vi "一体站流程质控自动启动.vi"(6 "CODMn量程切换":enum32{"H", "L", "AUTO"}(ring)=enum."AUTO", 8 "总磷量程切换":enum32{"H", "L", "AUTO"}(ring)=enum."AUTO", 9 "总氮量程切换":enum32{"H", "L", "AUTO"}(ring)=enum."AUTO", 10 "氨氮量程切换":enum32{"H", "L", "AUTO"}(ring)=enum."AUTO", 11 "参数":T1={"是否启用仪器"=FALSE, "CODMn"={"启动测量模式"={"测量模式"=enum."水样测量"}, "确定按钮"=TRUE}, "启动模块"={"氨氮"=FALSE, "总磷"=FALSE, "总氮"=FALSE, "COD"=FALSE}, "常规启动"=FALSE, "直接启动"=FALSE}) -> ()   [LabVIEW 2016, in "质控单元.lvlib"]
uses:
  PLC/PLC.lvlib
panel:
  out "枚举 2":enum16{"初始化", "采配水启动", "等待", "配水", "排水", "结束"}(ring)
  out "枚举":enum16{"初始化", "采配水启动", "等待", "配水", "排水", "结束"}(ring)
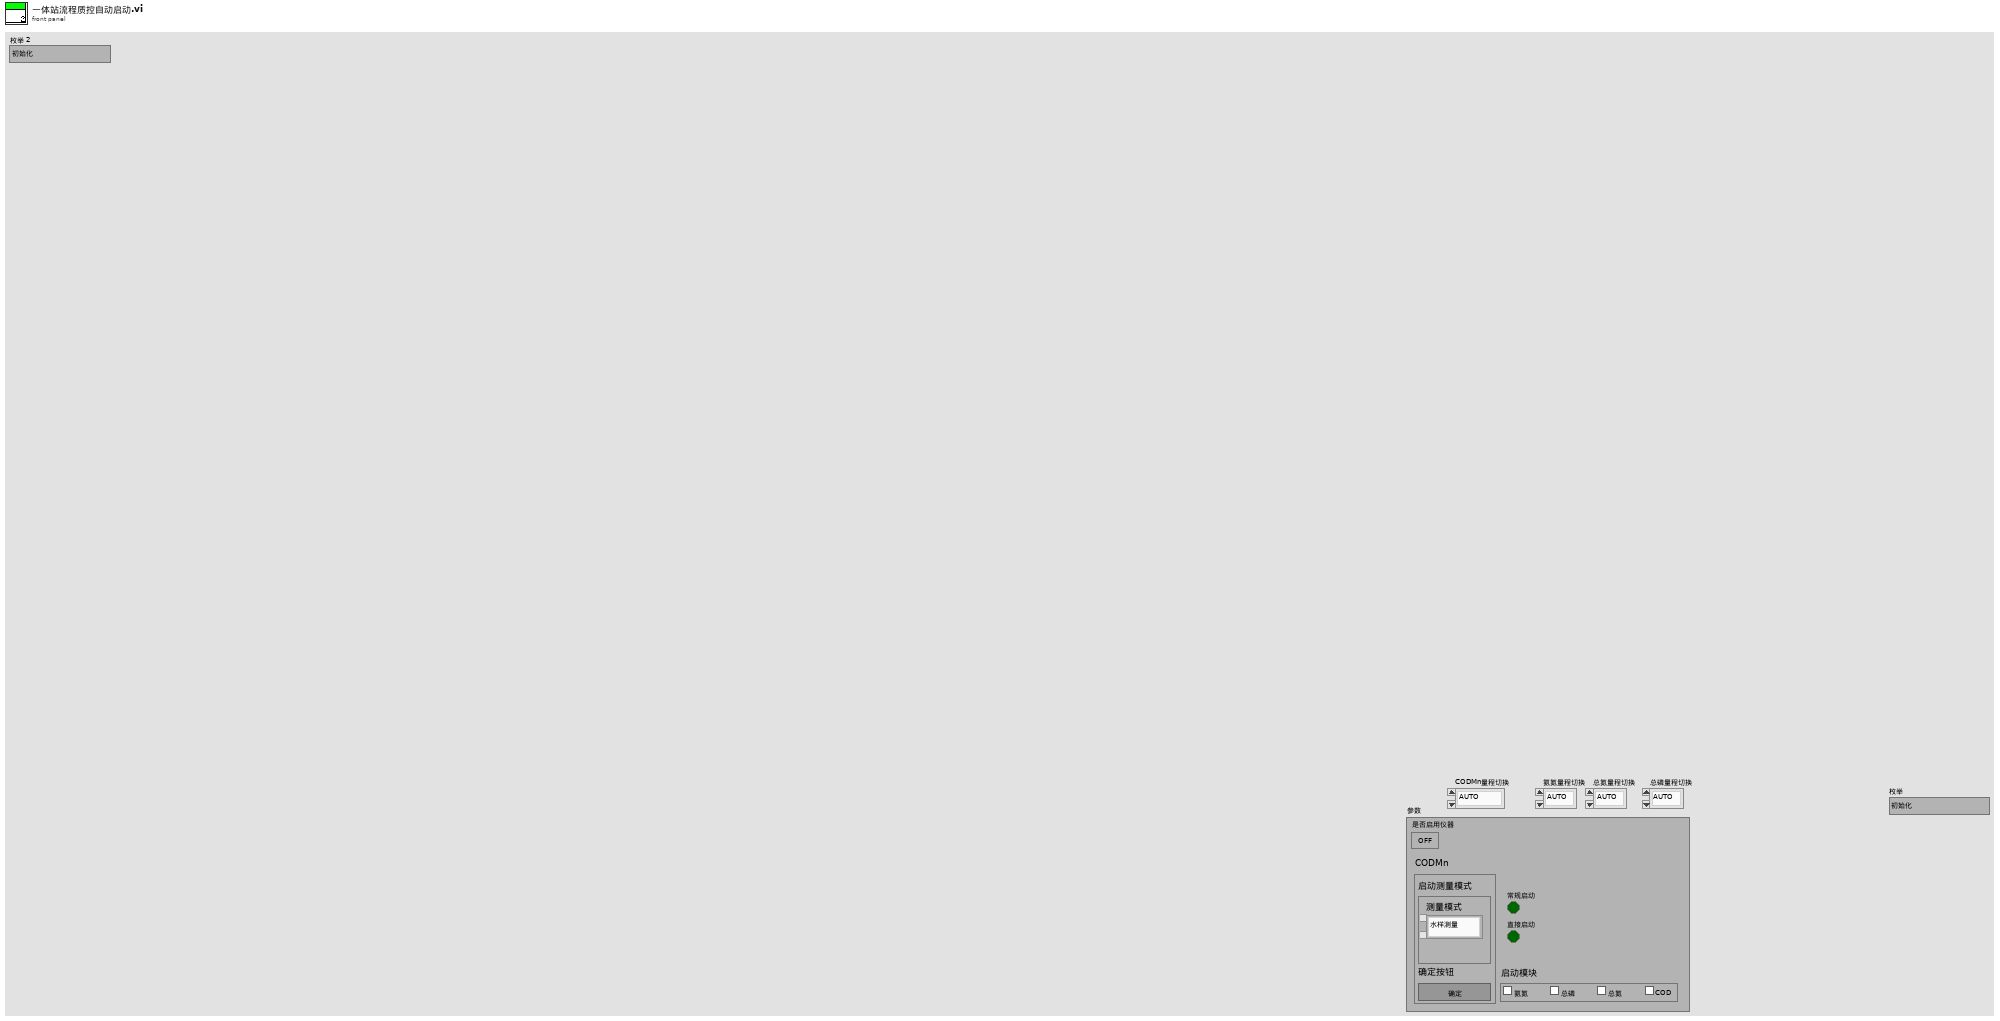
[diagram p1: front panel]
types:
  T1 = cluster{"是否启用仪器":bool, "CODMn":cluster{"启动测量模式":cluster{"测量模式":enum16{"水样测量", "标样核查", "加标回收", "平行样", "校零", "校标"}}, "确定按钮":bool}, "启动模块":cluster{"氨氮":bool, "总磷":bool, "总氮":bool, "COD":bool}, "常规启动":bool, "直接启动":bool}
  T2 = cluster{"命令":string, cluster{"starting address":u16, "holding register value":u16}}
  T3 = cluster{"R0":i16, "R1":i16, "R2":i16, "R3":i16, "R4":i16, "R5":i16, "R6":i16, "R7":i16, "R8":i16, "R9":i16, "R10":i16, "R11":i16, "R12":i16, "R13":i16, "R14":i16, "R15":i16, "R16":i16, "R17":i16, "R18":i16, "R19":i16, "R20":i16, "R21":i16, "R22":i16, "R23":i16, "R24":i16, "R25":i16, "R26":i16, "R27":i16, "R28":i16, "R29":i16, "R30":i16, "R31":i16, "R32":i16, "R33":i16, "R34":i16, "R35":i16, "R36":i16, "R37":i16, "R38":i16, "R39":i16, "R40":i16, "R41":i16, "R42":i16, "R43":i16, "R44":i16, "R45":i16, "R46":i16, "R47":i16, "R48":i16, "R49":i16, "R50":i16, "R51":i16, "R52":i16, "R53":i16, "R54":i16, "R55":i16, "R56":i16}
  T4 = enum32{"Bad", "Idle", "Run top level", "Running"}
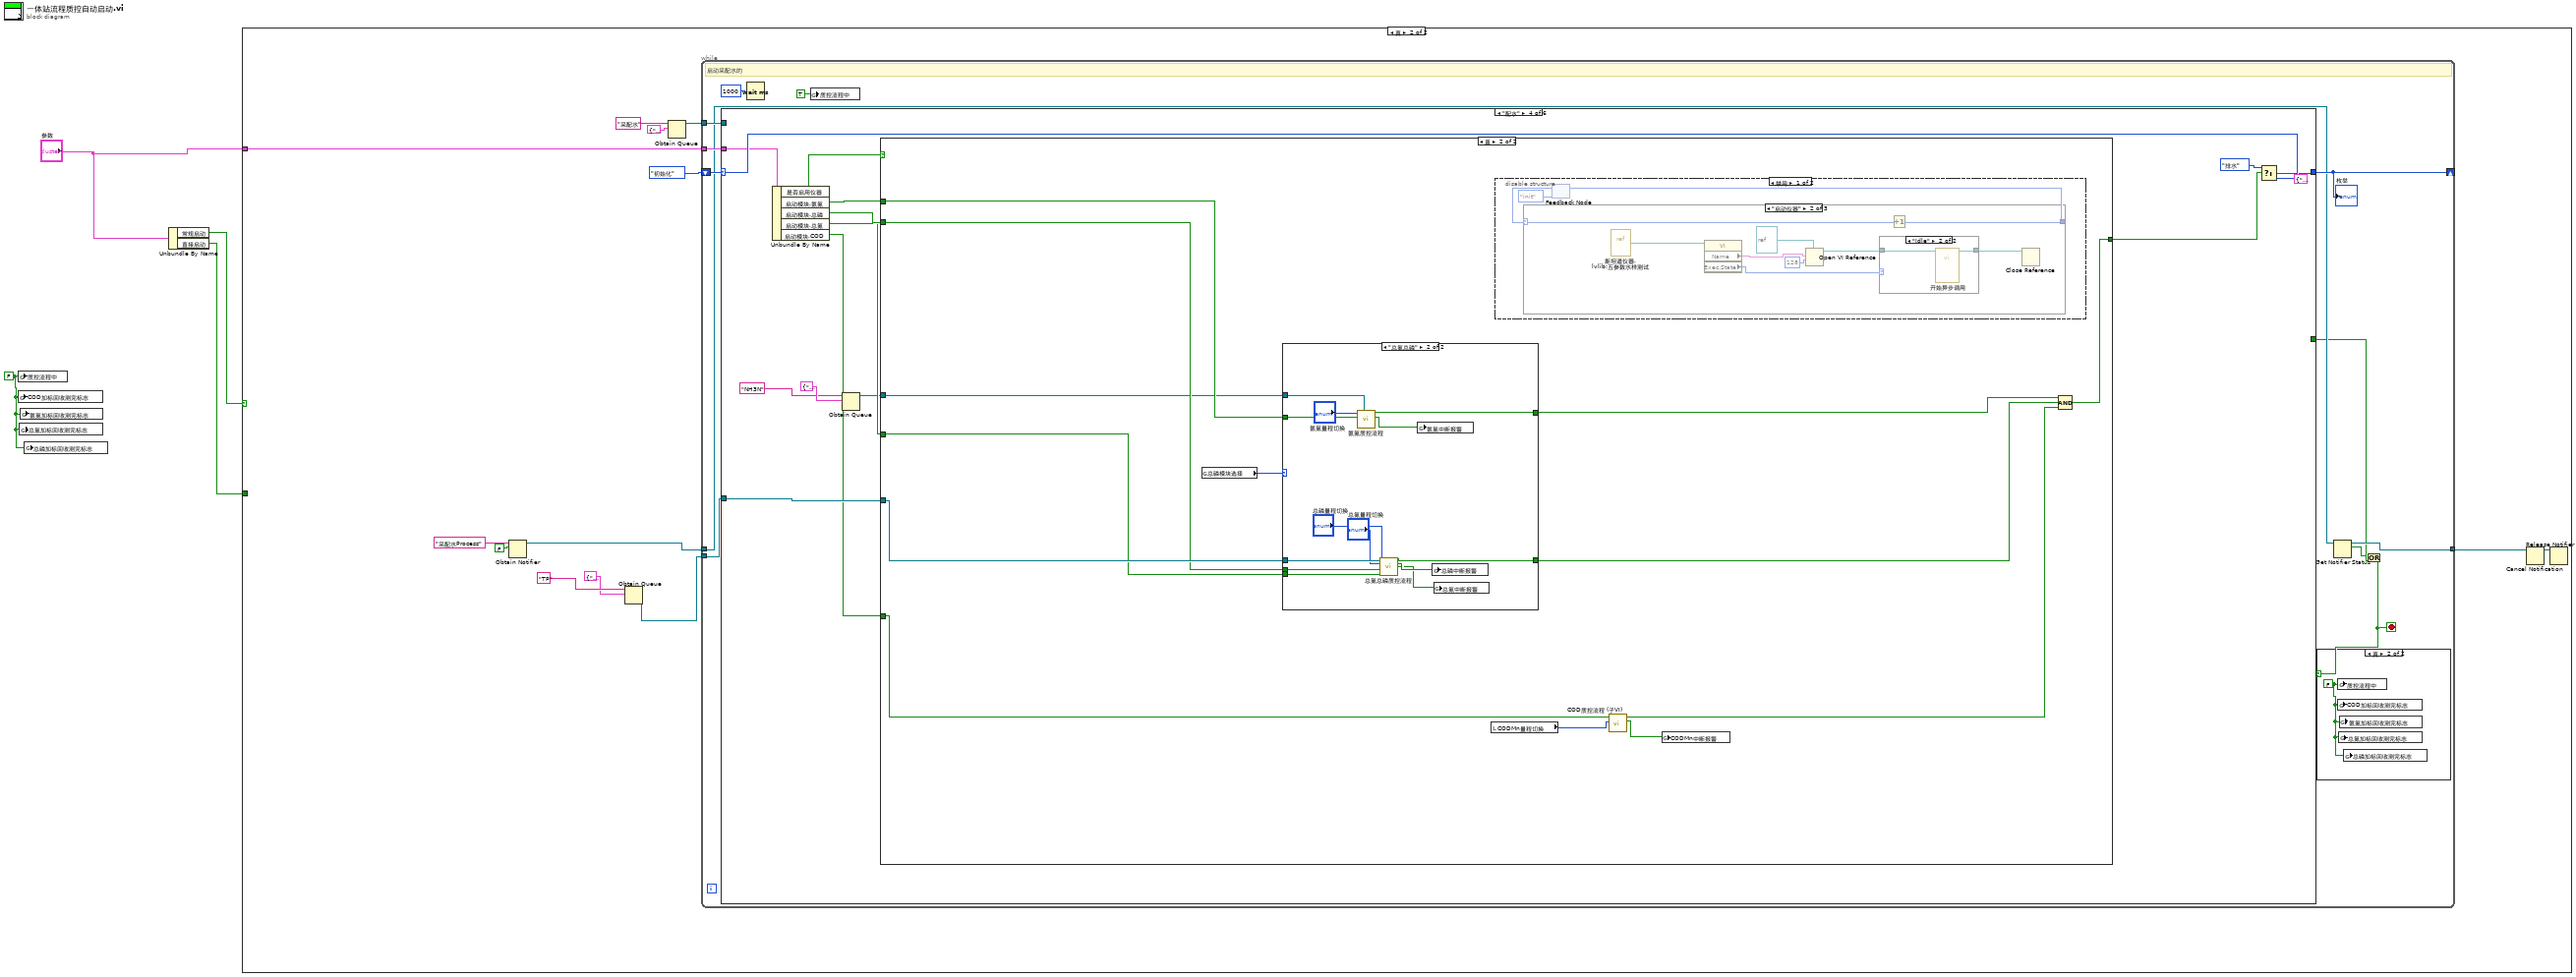
[diagram p0: block diagram]
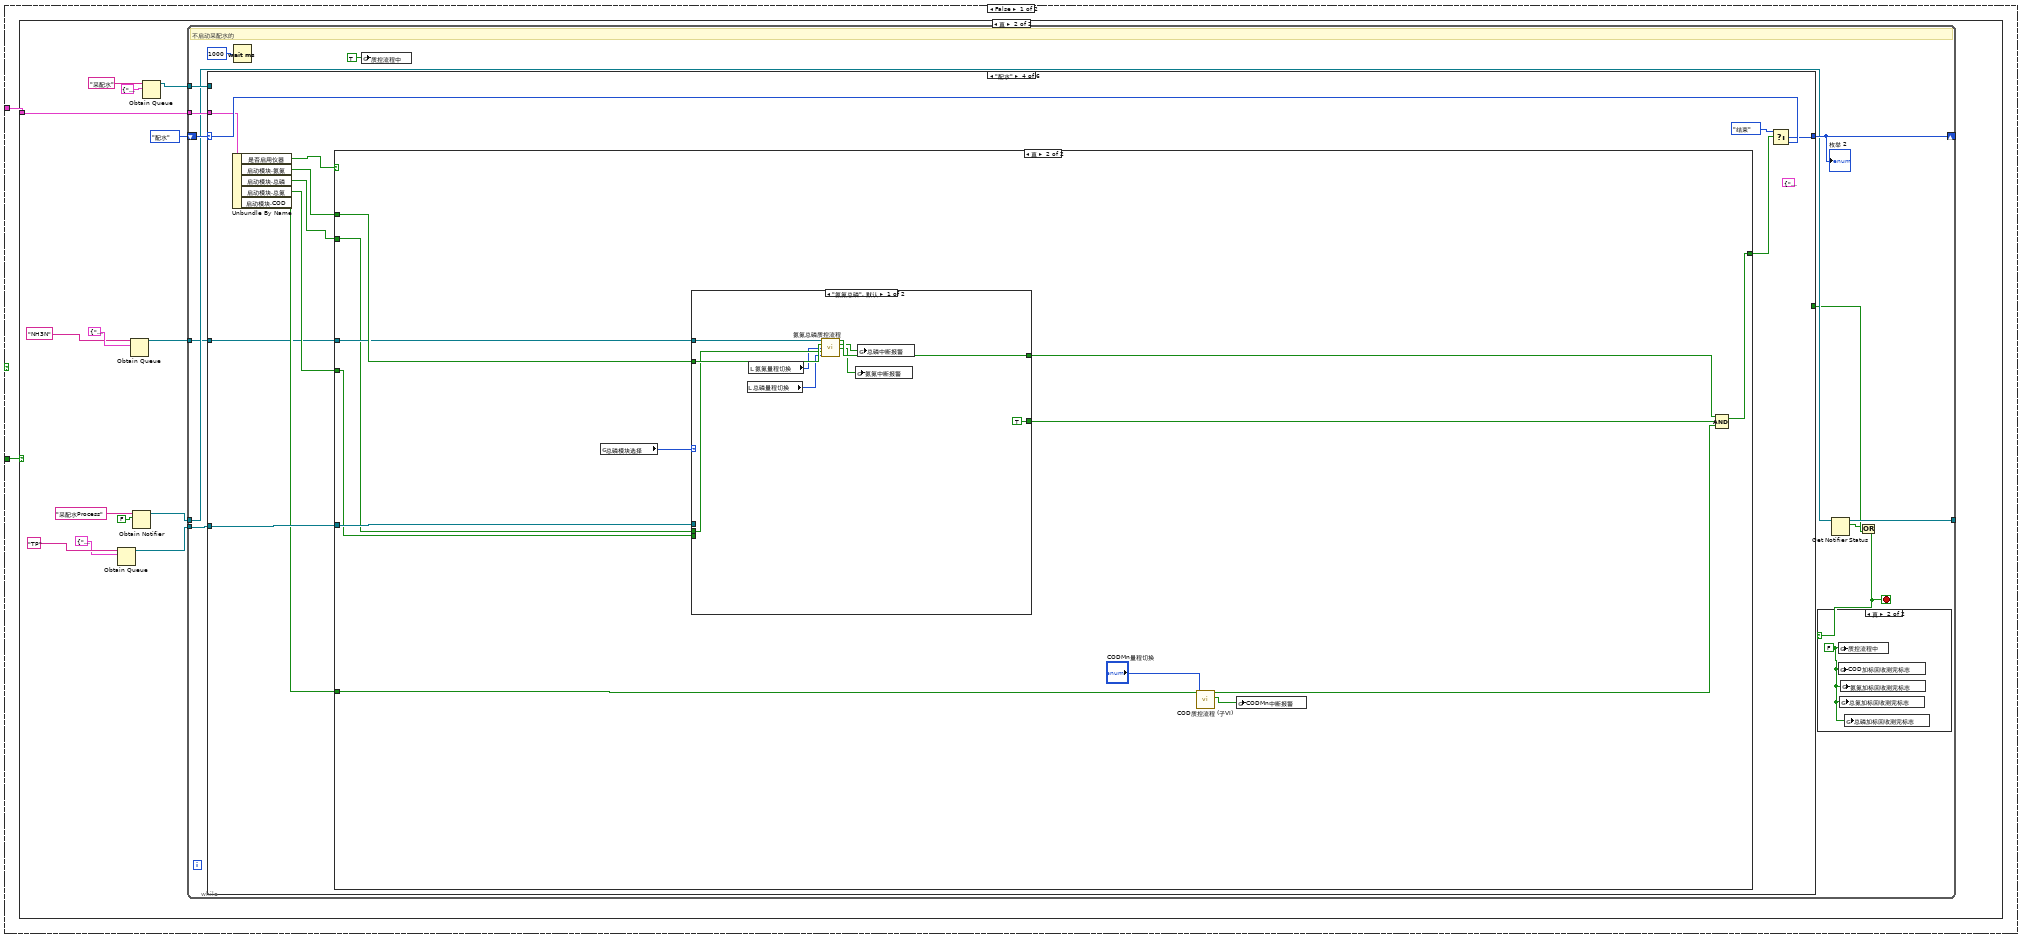
[diagram p2: hidden frame]
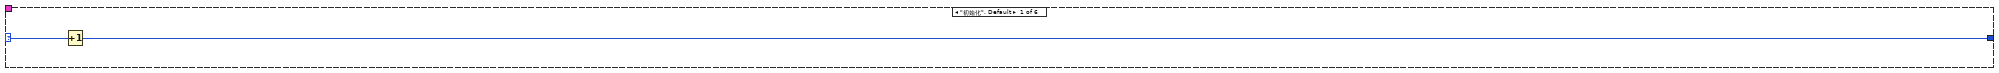
[diagram p5: hidden frame]
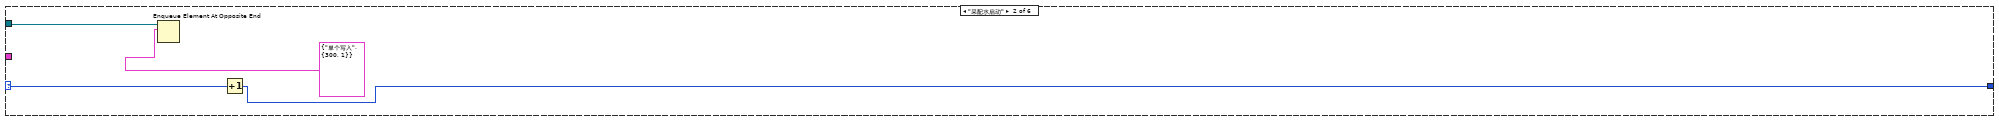
[diagram p6: hidden frame]
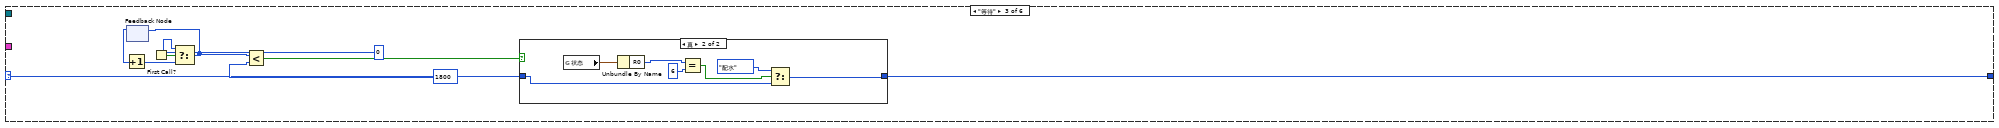
[diagram p7: hidden frame]
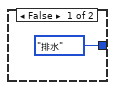
[diagram p8: hidden frame]
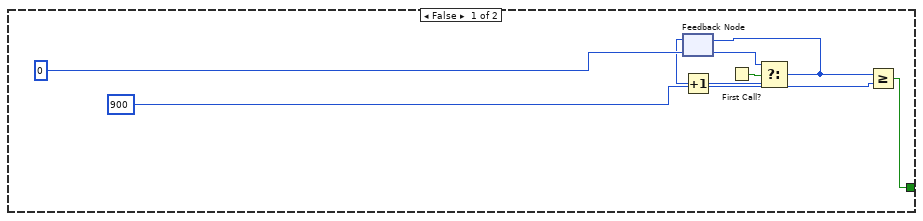
[diagram p9: hidden frame]
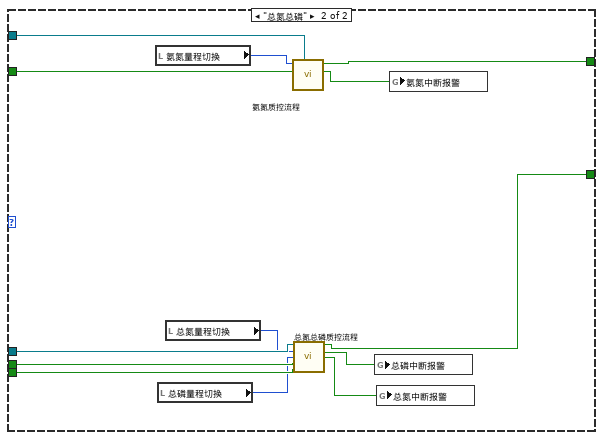
[diagram p10: hidden frame]
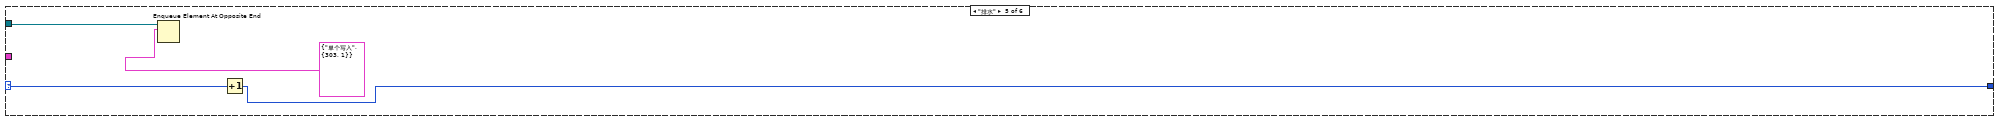
[diagram p11: hidden frame]
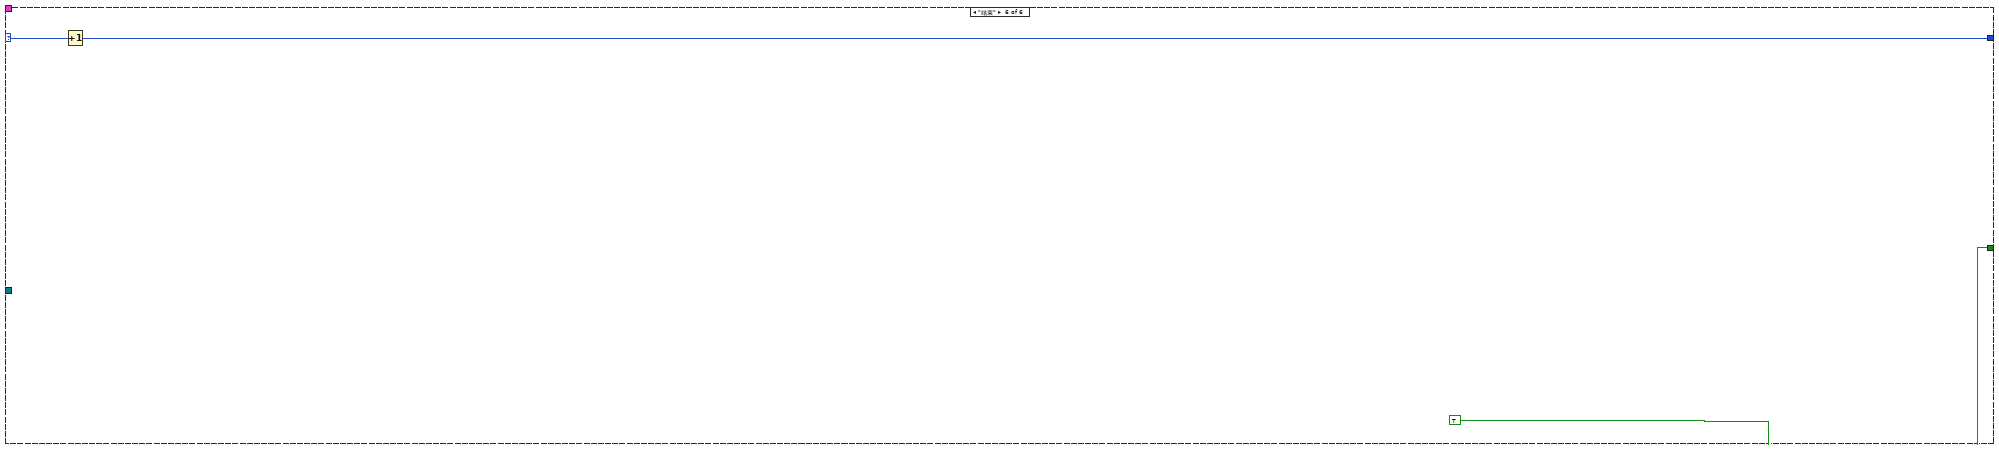
[diagram p12: hidden frame]
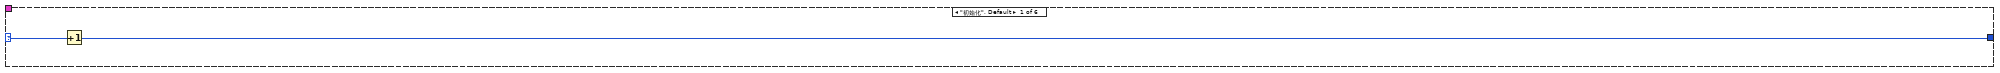
[diagram p14: hidden frame]
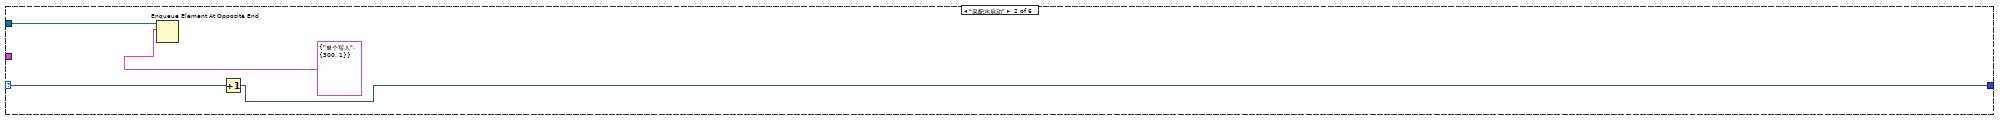
[diagram p15: hidden frame]
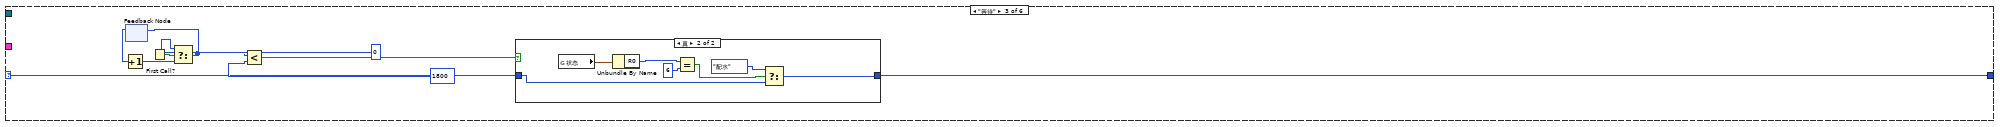
[diagram p16: hidden frame]
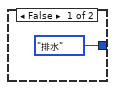
[diagram p17: hidden frame]
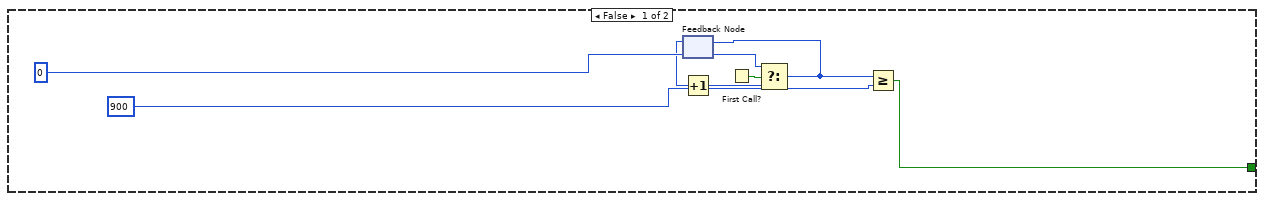
[diagram p18: hidden frame]
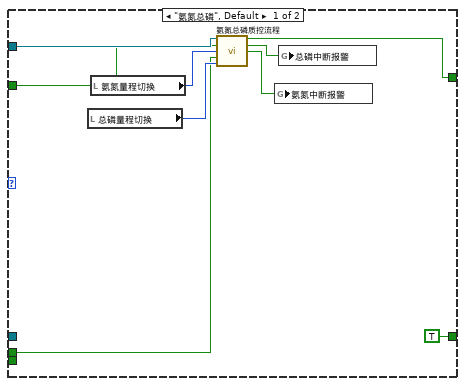
[diagram p19: hidden frame]
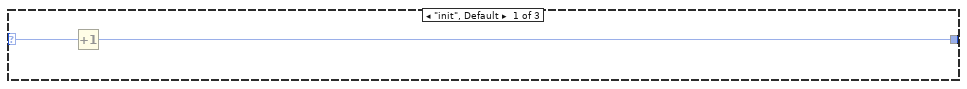
[diagram p20: hidden frame]
diagram:
  w1 = FALSE ("质控流程中")
  n1 = global write "质控测完标志全局 1.vi" "质控流程中"(w1) -> ()
  n2 = global write "质控测完标志全局 1.vi" "COD加标回收测完标志"(w1) -> ()
  n3 = global write "质控测完标志全局 1.vi" "总氮加标回收测完标志"(w1) -> ()
  n4 = global write "质控测完标志全局 1.vi" "氨氮加标回收测完标志"(w1) -> ()
  n5 = global write "质控测完标志全局 1.vi" "总磷加标回收测完标志"(w1) -> ()
  n6 = Unbundle By Name("参数") -> ("常规启动"=w3:bool, "直接启动"=w2:bool)
  n7 = case shown="真" w3 {
    tunnel: "参数" -> [w5 w119]
    tunnel: w2 -> [w6 _]
    frame False {
      n8 = case shown="真" w6 {
        tunnel: w5 -> [_ w19]
        frame False {
        }
        frame True {
          n9 = Obtain Queue(name (unnamed)="TP" ("名称（未命名）"), element data type=cluster{"命令":string, "data":variant} {"命令"="", "data"=variant}) -> (queue out=w10:refnum<queue>)  [unwired: 3 in, 2 out]
          n10 = Obtain Queue(name (unnamed)="NH3N" ("名称（未命名）"), element data type=cluster{"命令":string, "data":variant} {"命令"="", "data"=variant}) -> (queue out=w7:refnum<queue>)  [unwired: 3 in, 2 out]
          n11 = Obtain Notifier(name (unnamed)="采配水Process" ("名称（未命名）"), notification data type=FALSE) -> (notifier out=w13:refnum<notifier>)  [unwired: 2 in, 2 out]
          n12 = Obtain Queue(name (unnamed)="采配水" ("名称（未命名）"), element data type=cluster{"命令":string, "数据":variant} {"命令"="", "数据"=variant}) -> (queue out=w16:refnum<queue>)  [unwired: 3 in, 2 out]
          n13 = while {
            tunnel: w16 -> [w33]
            shift-right: [w31] -> _
            shift-left: enum16{"初始化", "采配水启动", "等待", "配水", "排水", "结束"}."配水" ("枚举") -> [w32]
            tunnel: w10 -> [w29]
            tunnel: w19 -> [w28]
            tunnel: w13 -> [w27]
            tunnel: [w26] -> _
            tunnel: w7 -> [w23]
            stop <- w22 stop-if-true
            # "不启动采配水的"
            n14 = case shown="\"配水\"" w32 {
              selector: w32 -> [w36 w38 w47 w68 w113 w118]
              tunnel: w33 -> [_ w39 _ _ w114 _]
              tunnel: [w35 w37 w46 w67 w112 w117] -> w31
              tunnel: [_ _ _ _ _ TRUE] -> w25
              tunnel: w29 -> [_ _ _ w66 _ _]
              tunnel: w28 -> [_ _ _ w63 _ _]
              tunnel: w23 -> [_ _ _ w58 _ _]
              frame "初始化", Default {
                n15 = Increment(x=w36) -> (x+1=w35:enum16{"初始化", "采配水启动", "等待", "配水", "排水", "结束"})
              }
              frame "采配水启动" {
                n16 = Enqueue Element At Opposite End(queue=w39, element=T2 {"命令"="单个写入", {"starting address"=300, "holding register value"=1}} ("元素")) -> ()  [unwired: 2 in, 3 out]
                n17 = Increment(x=w38) -> (x+1=w37:enum16{"初始化", "采配水启动", "等待", "配水", "排水", "结束"})
              }
              frame "等待" {
                n18 = feedback #1() -> (w43:i32)  [unwired: 1 in]
                n19 = Increment(x=w43) -> (x+1=w42:i32)
                n20 = First Call?() -> (First Call?: T/F=w44:bool)
                n21 = Select(t=0, s=w44, f=w42) -> (s? t:f=w41:i32)
                n22 = feedback-in #1(w41) -> ()
                n23 = Less?(x=w41, y=1800) -> (x < y?=w48:bool)
                n24 = case shown="真" w48 {
                  tunnel: w47 -> [_ w52]
                  tunnel: [enum16{"初始化", "采配水启动", "等待", "配水", "排水", "结束"}."排水" ("枚举") w51] -> w46
                  frame False {
                  }
                  frame True {
                    n25 = global read "采配水全局变量.vi" "状态"() -> (w57:T3)
                    n26 = Unbundle By Name(w57) -> ("R0"=w56:i16)
                    n27 = Equal?(x=w56, y=i16 6) -> (x = y?=w54:bool)
                    n28 = Select(t=enum16{"初始化", "采配水启动", "等待", "配水", "排水", "结束"}."配水" ("枚举"), s=w54, f=w52) -> (s? t:f=w51:enum16{"初始化", "采配水启动", "等待", "配水", "排水", "结束"})
                  }
                }
              }
              frame "配水" {
                (unwired) cluster{"命令":string, "data":variant} {"命令"="启动", "data"=variant(cluster{"站号":u16, "控制命令输出":u16[]} {"站号"=1, "控制命令输出"=[256, 0]})} ("元素")
                n29 = Unbundle By Name(w63) -> ("是否启用仪器"=w65:bool, "启动模块.氨氮"=w61:bool, "启动模块.总磷"=w62:bool, "启动模块.总氮"=w59:bool, "启动模块.COD"=w60:bool)
                n30 = case shown="真" w65 {
                  tunnel: w66 -> [_ w83]
                  tunnel: [w70 w89] -> w64
                  tunnel: w62 -> [_ w82]
                  tunnel: w61 -> [_ w88]
                  tunnel: w60 -> [_ w87]
                  tunnel: w59 -> [_ w81]
                  tunnel: w58 -> [_ w85]
                  frame False {
                    n31 = feedback #2() -> (w74:i32)  [unwired: 1 in]
                    n32 = Increment(x=w74) -> (x+1=w73:i32)
                    n33 = First Call?() -> (First Call?: T/F=w75:bool)
                    n34 = Select(t=0, s=w75, f=w73) -> (s? t:f=w71:i32)
                    n35 = feedback-in #2(w71) -> ()
                    n36 = Greater Or Equal?(x=w71, y=900) -> (x >= y?=w70:bool)
                  }
                  frame True {
                    n37 = global read "质控测完标志全局 1.vi" "总磷模块选择"() -> (w77:enum32{"氨氮总磷", "总氮总磷"})
                    n38 = case shown="\"氨氮总磷\", 默认" w77 {
                      tunnel: w88 -> [w96 w111]
                      tunnel: [w92 w110] -> w86
                      tunnel: w85 -> [w97 w109]
                      tunnel: w83 -> [_ w108]
                      tunnel: w82 -> [w95 w107]
                      tunnel: w81 -> [_ w106]
                      tunnel: [TRUE ("布尔") w105] -> w80
                      frame "氨氮总磷", Default {
                        n39 = local read "总磷量程切换"() -> (w93:enum32{"H", "L", "AUTO"})
                        n40 = local read "氨氮量程切换"() -> (w94:enum32{"H", "L", "AUTO"})
                        n41 = call "氨氮总磷质控流程.vi"("队列输入"=w97, "氨氮"=w96, "氨氮量程切换"=w94, "总磷"=w95, "总磷量程切换"=w93) -> ("布尔"=w92:bool, "总磷中断报警"=w91:bool, "氨氮中断报警"=w90:bool)  [unwired: 8 in]
                        n42 = global write "质控中断报警全局.vi" "氨氮中断报警"(w90) -> ()
                        n43 = global write "质控中断报警全局.vi" "总磷中断报警"(w91) -> ()
                      }
                      frame "总氮总磷" {
                        n44 = local read "氨氮量程切换"() -> (w102:enum32{"H", "L", "AUTO"})
                        n45 = local read "总磷量程切换"() -> (w104:enum32{"H", "L", "AUTO"})
                        n46 = local read "总氮量程切换"() -> (w103:enum32{"H", "L", "AUTO"})
                        n47 = call "氨氮质控流程.vi"("队列输入NH3"=w109, "氨氮"=w111, "氨氮量程切换"=w102) -> ("氨氮中断报警"=w101:bool, "布尔"=w110:bool)  [unwired: 7 in]
                        n48 = call "总氮总磷质控流程.vi"("队列输入TP"=w108, "总氮量程切换"=w103, "总磷量程切换"=w104, "总磷"=w107, "总氮"=w106) -> ("布尔"=w105:bool, "总磷中断报警"=w100:bool, "总氮中断报警"=w99:bool)  [unwired: 8 in]
                        n49 = global write "质控中断报警全局.vi" "总磷中断报警"(w100) -> ()
                        n50 = global write "质控中断报警全局.vi" "总氮中断报警"(w99) -> ()
                        n51 = global write "质控中断报警全局.vi" "氨氮中断报警"(w101) -> ()
                      }
                    }
                    n52 = call "COD质控流程 (子VI).vi"("CODMn量程切换"="CODMn量程切换", "COD"=w87) -> ("CODMn中断报警"=w78:bool, "布尔"=w84:bool)  [unwired: 8 in]
                    n53 = global write "质控中断报警全局.vi" "CODMn中断报警"(w78) -> ()
                    n54 = Compound Arithmetic op=AND ("复合运算")(w86, w80, w84) -> (w89:bool)
                  }
                }
                n55 = Select(t=enum16{"初始化", "采配水启动", "等待", "配水", "排水", "结束"}."结束" ("枚举"), s=w64, f=w68) -> (s? t:f=w67:enum16{"初始化", "采配水启动", "等待", "配水", "排水", "结束"})
              }
              frame "排水" {
                n56 = Enqueue Element At Opposite End(queue=w114, element=T2 {"命令"="单个写入", {"starting address"=303, "holding register value"=1}} ("元素")) -> ()  [unwired: 2 in, 3 out]
                n57 = Increment(x=w113) -> (x+1=w112:enum16{"初始化", "采配水启动", "等待", "配水", "排水", "结束"})
              }
              frame "结束" {
                n58 = Increment(x=w118) -> (x+1=w117:enum16{"初始化", "采配水启动", "等待", "配水", "排水", "结束"})
              }
            }
            "枚举 2" <- w31
            n59 = Wait (ms)(milliseconds to wait=u32 1000 ("等待时间（毫秒）")) -> ()  [unwired: 1 out]
            n60 = global write "质控测完标志全局 1.vi" "质控流程中"(TRUE ("质控流程中")) -> ()
            n61 = Get Notifier Status(notifier=w27) -> (notifier out=w26:refnum<notifier>, current notification=w24:bool)  [unwired: 1 in, 3 out]
            n62 = Or(x=w24, y=w25) -> (x .or. y?=w22:bool)
            n63 = case shown="真" w22 {
              frame False {
              }
              frame True {
                w34 = FALSE ("质控流程中")
                n64 = global write "质控测完标志全局 1.vi" "质控流程中"(w34) -> ()
                n65 = global write "质控测完标志全局 1.vi" "COD加标回收测完标志"(w34) -> ()
                n66 = global write "质控测完标志全局 1.vi" "总氮加标回收测完标志"(w34) -> ()
                n67 = global write "质控测完标志全局 1.vi" "氨氮加标回收测完标志"(w34) -> ()
                n68 = global write "质控测完标志全局 1.vi" "总磷加标回收测完标志"(w34) -> ()
              }
            }
          }
        }
      }
    }
    frame True {
      n69 = Obtain Notifier(name (unnamed)="采配水Process" ("名称（未命名）"), notification data type=FALSE) -> (notifier out=w122:refnum<notifier>)  [unwired: 2 in, 2 out]
      n70 = Obtain Queue(name (unnamed)="TP" ("名称（未命名）"), element data type=cluster{"命令":string, "data":variant} {"命令"="", "data"=variant}) -> (queue out=w125:refnum<queue>)  [unwired: 3 in, 2 out]
      n71 = Obtain Queue(name (unnamed)="采配水" ("名称（未命名）"), element data type=cluster{"命令":string, "数据":variant} {"命令"="", "数据"=variant}) -> (queue out=w129:refnum<queue>)  [unwired: 3 in, 2 out]
      n72 = while {
        tunnel: w129 -> [w143]
        shift-right: [w141] -> _
        shift-left: enum16{"初始化", "采配水启动", "等待", "配水", "排水", "结束"}."初始化" ("枚举") -> [w142]
        tunnel: w125 -> [w139]
        tunnel: w119 -> [w138]
        tunnel: w122 -> [w137]
        tunnel: [w136] -> w121
        stop <- w133 stop-if-true
        # "启动采配水的"
        n73 = case shown="\"配水\"" w142 {
          selector: w142 -> [w146 w148 w157 w180 w243 w248]
          tunnel: w143 -> [_ w149 _ _ w244 _]
          tunnel: [w145 w147 w156 w179 w242 w247] -> w141
          tunnel: [_ _ _ _ _ TRUE] -> w135
          tunnel: w139 -> [_ _ _ w178 _ _]
          tunnel: w138 -> [_ _ _ w175 _ _]
          frame "初始化", Default {
            n74 = Increment(x=w146) -> (x+1=w145:enum16{"初始化", "采配水启动", "等待", "配水", "排水", "结束"})
          }
          frame "采配水启动" {
            n75 = Enqueue Element At Opposite End(queue=w149, element=T2 {"命令"="单个写入", {"starting address"=300, "holding register value"=1}} ("元素")) -> ()  [unwired: 2 in, 3 out]
            n76 = Increment(x=w148) -> (x+1=w147:enum16{"初始化", "采配水启动", "等待", "配水", "排水", "结束"})
          }
          frame "等待" {
            n77 = feedback #3() -> (w153:i32)  [unwired: 1 in]
            n78 = Increment(x=w153) -> (x+1=w152:i32)
            n79 = First Call?() -> (First Call?: T/F=w154:bool)
            n80 = Select(t=0, s=w154, f=w152) -> (s? t:f=w151:i32)
            n81 = feedback-in #3(w151) -> ()
            n82 = Less?(x=w151, y=1800) -> (x < y?=w158:bool)
            n83 = case shown="真" w158 {
              tunnel: w157 -> [_ w162]
              tunnel: [enum16{"初始化", "采配水启动", "等待", "配水", "排水", "结束"}."排水" ("枚举") w161] -> w156
              frame False {
              }
              frame True {
                n84 = global read "采配水全局变量.vi" "状态"() -> (w167:T3)
                n85 = Unbundle By Name(w167) -> ("R0"=w166:i16)
                n86 = Equal?(x=w166, y=i16 6) -> (x = y?=w164:bool)
                n87 = Select(t=enum16{"初始化", "采配水启动", "等待", "配水", "排水", "结束"}."配水" ("枚举"), s=w164, f=w162) -> (s? t:f=w161:enum16{"初始化", "采配水启动", "等待", "配水", "排水", "结束"})
              }
            }
          }
          frame "配水" {
            (unwired) cluster{"命令":string, "data":variant} {"命令"="启动", "data"=variant(cluster{"站号":u16, "控制命令输出":u16[]} {"站号"=1, "控制命令输出"=[256, 0]})} ("元素")
            n88 = Unbundle By Name(w175) -> ("是否启用仪器"=w177:bool, "启动模块.氨氮"=w173:bool, "启动模块.总磷"=w174:bool, "启动模块.总氮"=w171:bool, "启动模块.COD"=w172:bool)
            n89 = Obtain Queue(name (unnamed)="NH3N" ("名称（未命名）"), element data type=cluster{"命令":string, "data":variant} {"命令"="", "data"=variant}) -> (queue out=w168:refnum<queue>)  [unwired: 3 in, 2 out]
            n90 = case shown="真" w177 {
              tunnel: w178 -> [_ w196]
              tunnel: [w182 w200] -> w176
              tunnel: w174 -> [_ w195]
              tunnel: w173 -> [_ w199]
              tunnel: w172 -> [_ w198]
              tunnel: w171 -> [_ w194]
              tunnel: w168 -> [_ w192]
              frame False {
                n91 = feedback #4() -> (w186:i32)  [unwired: 1 in]
                n92 = Increment(x=w186) -> (x+1=w185:i32)
                n93 = First Call?() -> (First Call?: T/F=w187:bool)
                n94 = Select(t=0, s=w187, f=w185) -> (s? t:f=w183:i32)
                n95 = feedback-in #4(w183) -> ()
                n96 = Greater Or Equal?(x=w183, y=900) -> (x >= y?=w182:bool)
              }
              frame True {
                n97 = global read "质控测完标志全局 1.vi" "总磷模块选择"() -> (w189:enum32{"氨氮总磷", "总氮总磷"})
                n98 = case shown="\"总氮总磷\"" w189 {
                  tunnel: [w203 w223] -> w201
                  tunnel: w199 -> [w205 w222]
                  tunnel: w196 -> [_ w221]
                  tunnel: w195 -> [w204 w220]
                  tunnel: w194 -> [_ w219]
                  tunnel: [TRUE ("布尔") w218] -> w193
                  tunnel: w192 -> [w206 w215]
                  frame "氨氮总磷", Default {
                    n99 = local read "总磷量程切换"() -> (w209:enum32{"H", "L", "AUTO"})
                    n100 = local read "氨氮量程切换"() -> (w210:enum32{"H", "L", "AUTO"})
                    n101 = call "氨氮总磷质控流程.vi"("队列输入"=w206, "氨氮"=w205, "氨氮量程切换"=w210, "总磷"=w204, "总磷量程切换"=w209) -> ("布尔"=w203:bool, "总磷中断报警"=w208:bool, "氨氮中断报警"=w207:bool)  [unwired: 8 in]
                    n102 = global write "质控中断报警全局.vi" "氨氮中断报警"(w207) -> ()
                    n103 = global write "质控中断报警全局.vi" "总磷中断报警"(w208) -> ()
                  }
                  frame "总氮总磷" {
                    n104 = call "氨氮质控流程.vi"("队列输入NH3"=w215, "氨氮"=w222, "氨氮量程切换"="氨氮量程切换") -> ("氨氮中断报警"=w211:bool, "布尔"=w223:bool)  [unwired: 7 in]
                    n105 = call "总氮总磷质控流程.vi"("队列输入TP"=w221, "总氮量程切换"="总氮量程切换", "总磷量程切换"="总磷量程切换", "总磷"=w220, "总氮"=w219) -> ("布尔"=w218:bool, "总磷中断报警"=w213:bool, "总氮中断报警"=w212:bool)  [unwired: 8 in]
                    n106 = global write "质控中断报警全局.vi" "氨氮中断报警"(w211) -> ()
                    n107 = global write "质控中断报警全局.vi" "总磷中断报警"(w213) -> ()
                    n108 = global write "质控中断报警全局.vi" "总氮中断报警"(w212) -> ()
                  }
                }
                n109 = local read "CODMn量程切换"() -> (w191:enum32{"H", "L", "AUTO"})
                n110 = disable-structure shown="禁用" {
                  frame Disabled {
                    n111 = feedback #5(enum16{"init", "启动仪器", "测量中"}."init") -> (w225:enum16{"init", "启动仪器", "测量中"})
                    n112 = case shown="\"启动仪器\"" w225 {
                      selector: w225 -> [w228 w237 _]
                      tunnel: [w227 w236 enum16{"init", "启动仪器", "测量中"}."测量中"] -> w226
                      frame "init", Default {
                        n113 = Increment(x=w228) -> (x+1=w227:enum16{"init", "启动仪器", "测量中"})
                      }
                      frame "启动仪器" {
                        n114 = vi-ref "斯坦道仪器.lvlib:五参数水样测试.vi"() -> (w229:refnum<vi>)
                        n115 = property class="VI"(reference=w229) -> ("Name"=w233:string, "Exec.State"=w231:T4)  [unwired: 1 in, 2 out]
                        n116 = Open VI Reference(type specifier VI Refnum (for type only)=refnum<vi> refnum ("类型说明符VI引用句柄（仅用于类型）"), vi path=w233, options=128 ("选项")) -> (vi reference=w232:refnum<vi>)  [unwired: 3 in, 1 out]
                        n117 = case shown="\"Idle\"" w231 {
                          tunnel: w232 -> [w238 w240]
                          tunnel: [w238 w239] -> w230
                          frame "Bad", Default {
                          }
                          frame "Idle" {
                            n118 = call-by-ref "开始异步调用"(reference=w240) -> (reference out=w239:refnum<vi>)  [unwired: 13 in, 1 out]
                          }
                        }
                        n119 = Increment(x=w237) -> (x+1=w236:enum16{"init", "启动仪器", "测量中"})
                        n120 = Close Reference(reference=w230) -> ()  [unwired: 1 in, 1 out]
                      }
                      frame "测量中" {
                      }
                    }
                    n121 = feedback-in #5(w226) -> ()
                  }
                  frame Enabled {
                  }
                }
                n122 = call "COD质控流程 (子VI).vi"("CODMn量程切换"=w191, "COD"=w198) -> ("CODMn中断报警"=w190:bool, "布尔"=w197:bool)  [unwired: 8 in]
                n123 = global write "质控中断报警全局.vi" "CODMn中断报警"(w190) -> ()
                n124 = Compound Arithmetic op=AND ("复合运算")(w201, w193, w197) -> (w200:bool)
              }
            }
            n125 = Select(t=enum16{"初始化", "采配水启动", "等待", "配水", "排水", "结束"}."排水" ("枚举"), s=w176, f=w180) -> (s? t:f=w179:enum16{"初始化", "采配水启动", "等待", "配水", "排水", "结束"})
          }
          frame "排水" {
            n126 = Enqueue Element At Opposite End(queue=w244, element=T2 {"命令"="单个写入", {"starting address"=303, "holding register value"=1}} ("元素")) -> ()  [unwired: 2 in, 3 out]
            n127 = Increment(x=w243) -> (x+1=w242:enum16{"初始化", "采配水启动", "等待", "配水", "排水", "结束"})
          }
          frame "结束" {
            n128 = Increment(x=w248) -> (x+1=w247:enum16{"初始化", "采配水启动", "等待", "配水", "排水", "结束"})
          }
        }
        "枚举" <- w141
        n129 = Wait (ms)(milliseconds to wait=u32 1000 ("等待时间（毫秒）")) -> ()  [unwired: 1 out]
        n130 = global write "质控测完标志全局 1.vi" "质控流程中"(TRUE ("质控流程中")) -> ()
        n131 = Get Notifier Status(notifier=w137) -> (notifier out=w136:refnum<notifier>, current notification=w134:bool)  [unwired: 1 in, 3 out]
        n132 = Or(x=w134, y=w135) -> (x .or. y?=w133:bool)
        n133 = case shown="真" w133 {
          frame False {
          }
          frame True {
            w144 = FALSE ("质控流程中")
            n134 = global write "质控测完标志全局 1.vi" "质控流程中"(w144) -> ()
            n135 = global write "质控测完标志全局 1.vi" "COD加标回收测完标志"(w144) -> ()
            n136 = global write "质控测完标志全局 1.vi" "总氮加标回收测完标志"(w144) -> ()
            n137 = global write "质控测完标志全局 1.vi" "氨氮加标回收测完标志"(w144) -> ()
            n138 = global write "质控测完标志全局 1.vi" "总磷加标回收测完标志"(w144) -> ()
          }
        }
      }
      n139 = Cancel Notification(0:w121) -> (8:w120:refnum<notifier>)  [unwired: 1 in, 2 out]
      n140 = Release Notifier(notifier=w120) -> ()  [unwired: 2 in, 3 out]
    }
  }
